vi "get_LM_states_by_name.vi"(8 "error in (no error)":errorcluster caption="错误输入（无错误）", 10 "name":string, 11 "MotorSystem 输入":refnum<class "MotorSystem.lvclass">) -> (0 "error out":errorcluster caption="错误输出", 2 "簇":cluster{"state -":bool, "state +":bool}, 3 "MotorSystem 输出":refnum<class "MotorSystem.lvclass">)   [LabVIEW 2016, in "MotionControl_UFO_3DOF.lvlib" / "MotorSystem.lvclass"]
uses:
  <userlib>/MotionControl_UFO_3DOF/MotorSystem/MotorSystem.lvclass
  <userlib>/MotionControl_UFO_3DOF/MotorSystem/MotorSystem.lvclass/MotorSystem.ctl
  <userlib>/MotionControl_UFO_3DOF/OneMotion/OneMotion.lvclass/OneMotion.ctl
  <userlib>/MotionControl_UFO_3DOF/LimitSwitch/LimitSwitch.lvclass/LimitSwitch.ctl
  <userlib>/UISimCanFunc_wrapper/VIs/sensor/Uim SFBK wrapper.vi
  <userlib>/MotionControl_UFO_3DOF/OneMotion/OneMotion.lvclass
  <userlib>/MotionControl_UFO_3DOF/LimitSwitch/LimitSwitch.lvclass
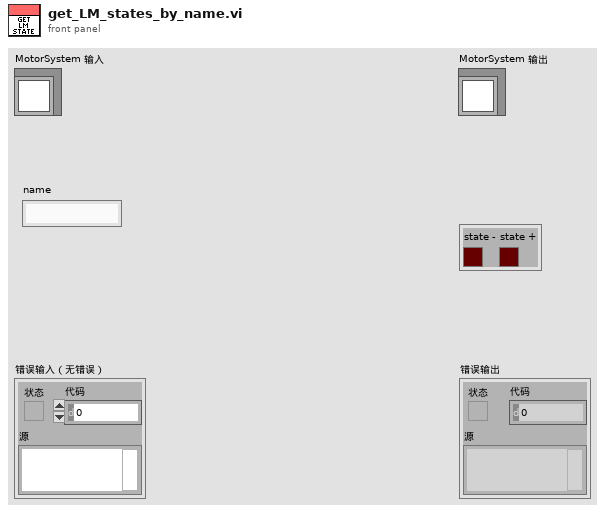
[diagram p1: front panel]
types:
  T1 = typedef "MotionControl_UFO_3DOF.lvlib/MotorSystem.lvclass/MotionCluster.ctl" = cluster{"OneMotion.lvclass":refnum<class "OneMotion.lvclass">, "connected?":bool, "default enabled?":bool, "enabled?":bool}
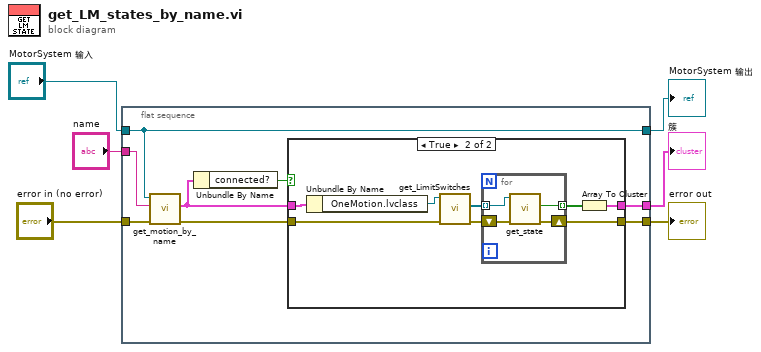
[diagram p0: block diagram]
diagram:
  n1 = flat-sequence {
    tunnel: [w10] -> w6
    tunnel: [w14] -> w4
    tunnel: "MotorSystem 输入" -> [w14]
    tunnel: "error in (no error)" -> [w12]
    tunnel: [w9] -> w1
    tunnel: "name" -> [w13]
    frame #0 {
      n2 = call <userlib>:"get_motion_by_name.vi"("error in (no error)"=w12, "name"=w13, "MotorSystem in"=w14) -> ("error out"=w11:errorcluster, "motion cluster"=w8:T1)  [unwired: 6 in, 1 out]
      n3 = Unbundle By Name(w8) -> ("connected?"=w7:bool)
      n4 = case shown="True" w7 {
        tunnel: w11 -> [w15 w23]
        tunnel: w8 -> [_ w20]
        tunnel: [w15 w18] -> w10
        tunnel: [_ w16] -> w9
        frame False {
        }
        frame True {
          n5 = Unbundle By Name(w20) -> ("OneMotion.lvclass"=w22:refnum<class "OneMotion.lvclass">)
          n6 = call <userlib>:"get_LimitSwitches.vi"("error in (no error)"=w23, "OneMotion输入"=w22) -> ("error out"=w21:errorcluster, "LimitSwitches"=w19:refnum<class "LimitSwitch.lvclass">[])  [unwired: 7 in, 1 out]
          n7 = for {
            tunnel: [w27] -> w17 mode=indexing
            shift-right: [w25] -> w18
            shift-left: w21 -> [w26]
            tunnel: w19 -> [w24] mode=indexing
            n8 = call <userlib>:"get_state.vi"("error in (no error)"=w26, "LimitSwitch输入"=w24) -> ("error out"=w25:errorcluster, "state"=w27:bool)  [unwired: 7 in, 1 out]
          }
          n9 = Array To Cluster(array=w17) -> (cluster=w16:cluster{"[0]":bool, "[1]":bool})
        }
      }
    }
  }
  "error out" <- w6
  "MotorSystem 输出" <- w4
  "簇" <- w1
